vi "Config_SaveKeys.vi"(8 "error in (no error)":errorcluster, 9 "Configuration Save":T1={"General"={"Config.ini"=path "", "Default Logging Path"=path ""}, "Hardware"={"AHC VISA COM"="", "Measure Rate (1/s)"=0, "Global T VAR"="", "Global B VAR"="", "Average"=4, "Bias"=0, "Cable"={"Length"=0.0, "Resistance"=0.0, "Inductance"=0.0, "Capacitance"=0.0}, "Tracking"=0, "Voltage"=0.0}, "Operation"={"Operation Mode"=enum."Idle-Off", "Status"="", "NewLog?"=FALSE}}, 10 "Configuration Cluster":T1={"General"={"Config.ini"=path "", "Default Logging Path"=path ""}, "Hardware"={"AHC VISA COM"="", "Measure Rate (1/s)"=0, "Global T VAR"="", "Global B VAR"="", "Average"=4, "Bias"=0, "Cable"={"Length"=0.0, "Resistance"=0.0, "Inductance"=0.0, "Capacitance"=0.0}, "Tracking"=0, "Voltage"=0.0}, "Operation"={"Operation Mode"=enum."Idle-Off", "Status"="", "NewLog?"=FALSE}}, 11 "Config In":T3) -> (0 "error out":errorcluster, 2 "output cluster":T1={"General"={"Config.ini"=path "", "Default Logging Path"=path ""}, "Hardware"={"AHC VISA COM"="", "Measure Rate (1/s)"=0, "Global T VAR"="", "Global B VAR"="", "Average"=4, "Bias"=0, "Cable"={"Length"=0.0, "Resistance"=0.0, "Inductance"=0.0, "Capacitance"=0.0}, "Tracking"=0, "Voltage"=0.0}, "Operation"={"Operation Mode"=enum."Idle-Off", "Status"="", "NewLog?"=FALSE}}, 3 "refnum out":T3)   [LabVIEW 2021]
uses:
  <vilib>/Utility/config.llb/Config Data RefNum.ctl
  Config_Cluster.ctl
  Mode_Enum.ctl
  <vilib>/Utility/config.llb/Write Key (Path).vi
  <vilib>/Utility/config.llb/Write Key (String).vi
  <vilib>/Utility/config.llb/Write Key (U32).vi
  <vilib>/Utility/config.llb/Write Key (Double).vi
  <vilib>/Utility/config.llb/Write Key (I32).vi
  <vilib>/Utility/config.llb/NI_LVConfig.lvlib
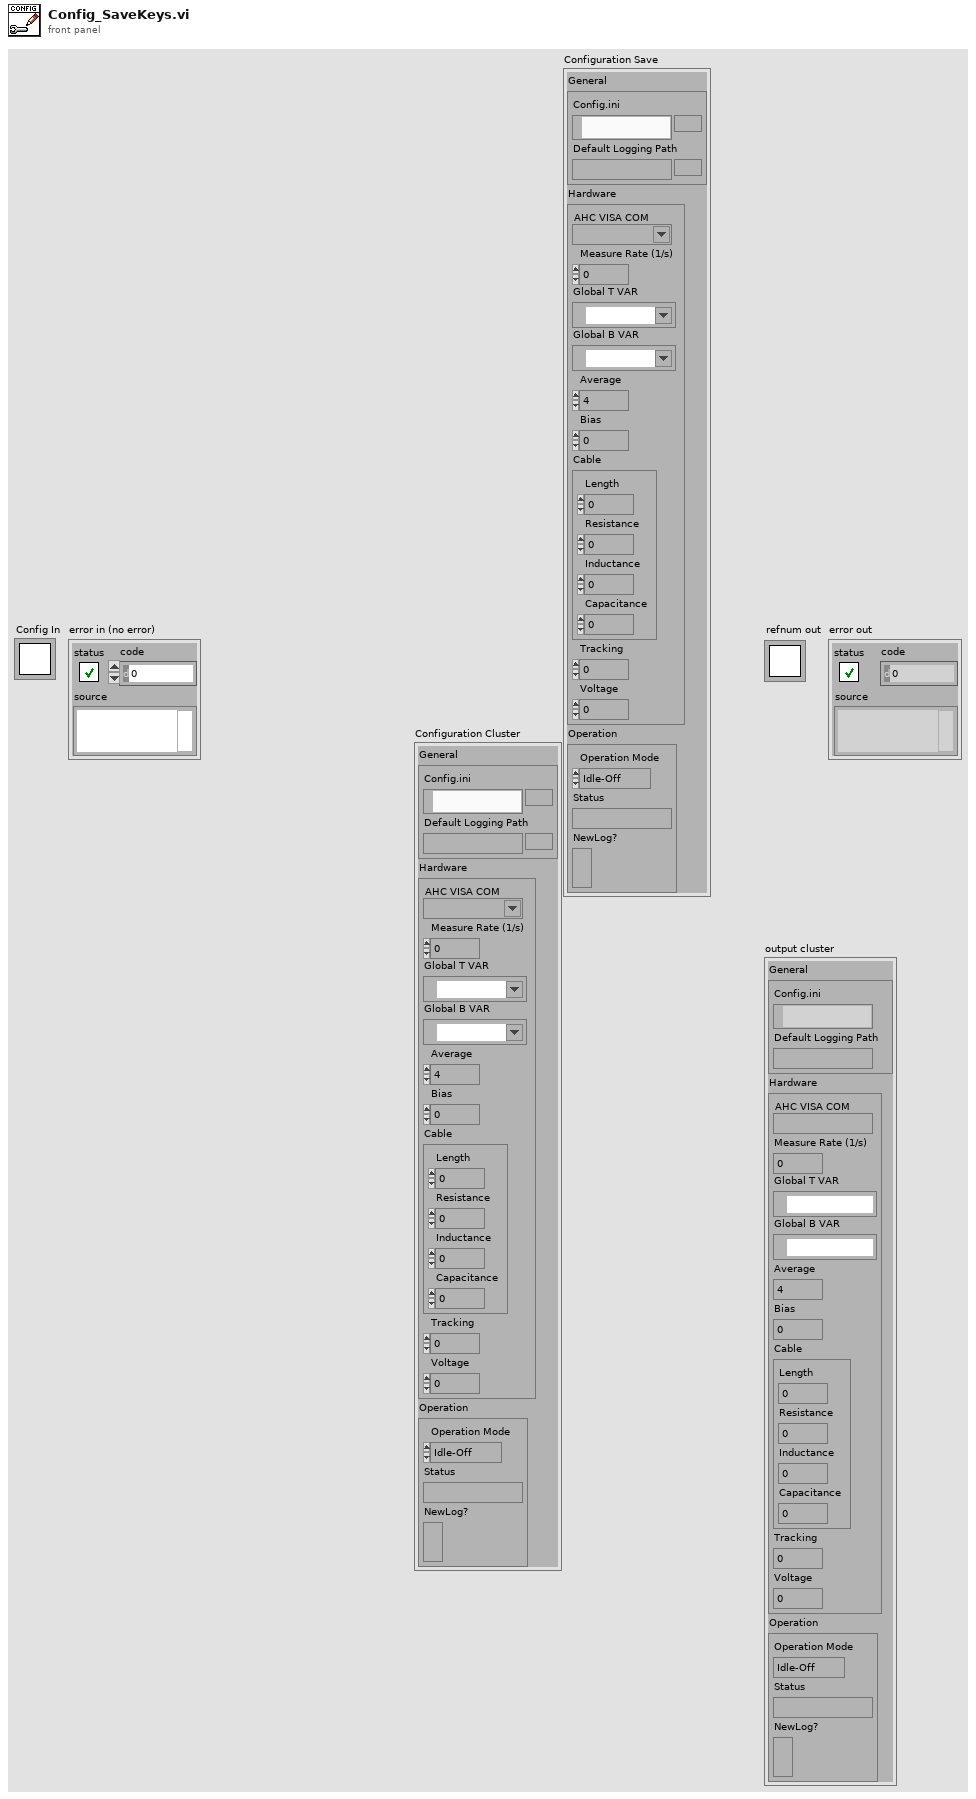
[diagram p1: front panel]
types:
  T1 = typedef "Config_Cluster.ctl" = cluster{"General":cluster{"Config.ini":path, "Default Logging Path":path}, "Hardware":cluster{"AHC VISA COM":refnum<visa-resource-name>, "Measure Rate (1/s)":i32, "Global T VAR":refnum<k21>, "Global B VAR":refnum<k21>, "Average":u8, "Bias":u8, "Cable":cluster{"Length":dbl, "Resistance":dbl, "Inductance":dbl, "Capacitance":dbl}, "Tracking":u8, "Voltage":dbl}, "Operation":cluster{"Operation Mode":T2, "Status":string, "NewLog?":bool}}
  T2 = typedef "Mode_Enum.ctl" = enum16{"Logging", "Idle-Off", "Idle"}
  T3 = typedef "NI_LVConfig.lvlib/Config Data RefNum.ctl" = refnum<k1>
  T4 = cluster{"Length":dbl, "Resistance":dbl, "Inductance":dbl, "Capacitance":dbl}
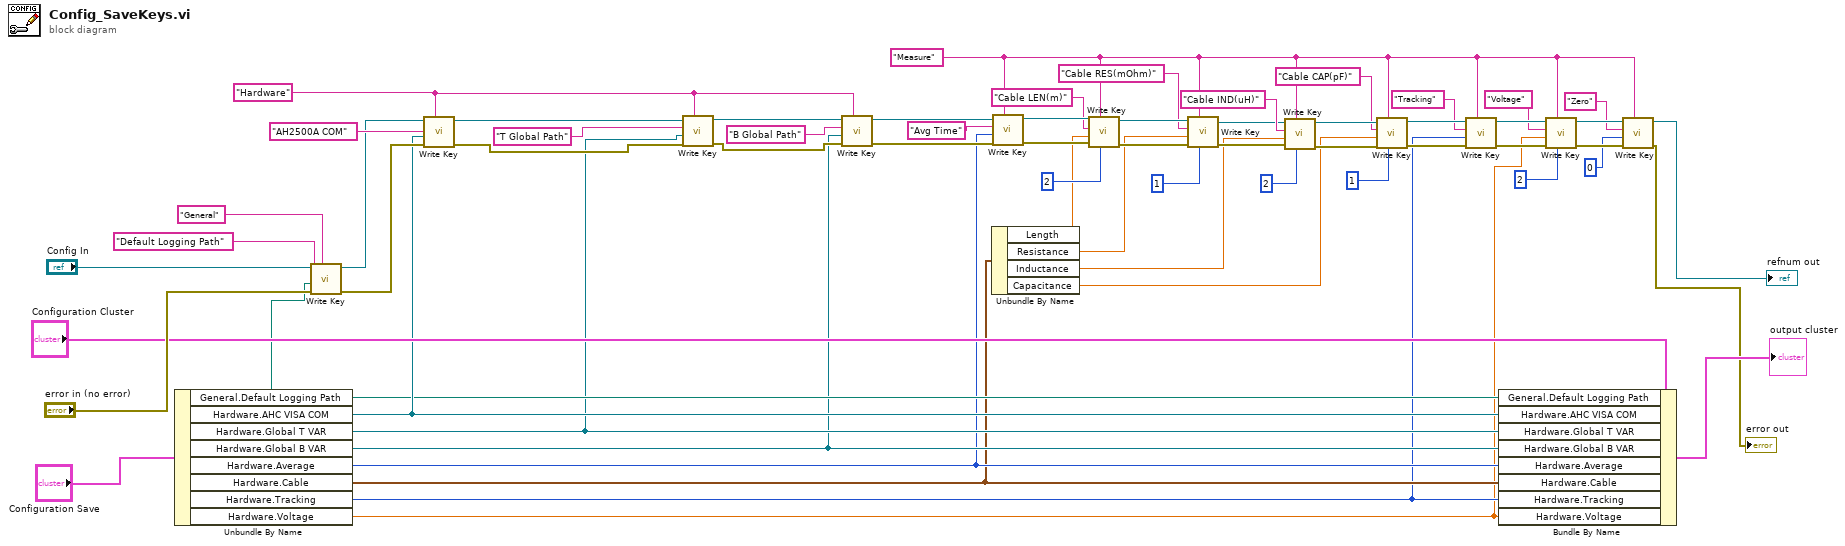
[diagram p0: block diagram]
diagram:
  w21 = "Measure" ("section")
  w52 = "Hardware" ("section")
  n1 = Unbundle By Name("Configuration Save") -> ("General.Default Logging Path"=w13:path, "Hardware.AHC VISA COM"=w14:refnum<visa-resource-name>, "Hardware.Global T VAR"=w12:refnum<k21>, "Hardware.Global B VAR"=w11:refnum<k21>, "Hardware.Average"=w10:u8, "Hardware.Cable"=w9:T4, "Hardware.Tracking"=w4:u8, "Hardware.Voltage"=w3:dbl)
  n2 = call-poly <vilib>:"Write Key.vi"("section"="General", "error in (no error)"="error in (no error)", "value"=w13, "key"="Default Logging Path", "refnum"="Config In") -> ("error out"=w16:errorcluster, "refnum out"=w17:T3)  [unwired: 4 in, 1 out]
  n3 = call-poly <vilib>:"Write Key.vi"("section"=w52, "error in (no error)"=w16, "value"=w14, "key"="AH2500A COM", "refnum"=w17) -> ("error out"=w54:errorcluster, "refnum out"=w55:T3)  [unwired: 4 in, 1 out]
  n4 = call-poly <vilib>:"Write Key.vi"("section"=w52, "error in (no error)"=w54, "value"=w12, "key"="T Global Path", "refnum"=w55) -> ("error out"=w49:errorcluster, "refnum out"=w53:T3)  [unwired: 4 in, 1 out]
  n5 = call-poly <vilib>:"Write Key.vi"("section"=w52, "error in (no error)"=w49, "value"=w11, "key"="B Global Path", "refnum"=w53) -> ("error out"=w47:errorcluster, "refnum out"=w48:T3)  [unwired: 4 in, 1 out]
  n6 = Unbundle By Name(w9) -> ("Length"=w8:dbl, "Resistance"=w7:dbl, "Inductance"=w6:dbl, "Capacitance"=w5:dbl)
  n7 = call-poly <vilib>:"Write Key.vi"("section"=w21, "error in (no error)"=w47, "value"=w10, "key"="Avg Time", "refnum"=w48) -> ("error out"=w44:errorcluster, "refnum out"=w45:T3)  [unwired: 4 in, 1 out]
  n8 = call-poly <vilib>:"Write Key.vi"("precision (6)"=i16 2, "section"=w21, "error in (no error)"=w44, "value"=w8, "key"="Cable LEN(m)", "refnum"=w45) -> ("error out"=w40:errorcluster, "refnum out"=w41:T3)  [unwired: 3 in, 1 out]
  n9 = call-poly <vilib>:"Write Key.vi"("precision (6)"=i16 1, "section"=w21, "error in (no error)"=w40, "value"=w7, "key"="Cable RES(mOhm)", "refnum"=w41) -> ("error out"=w36:errorcluster, "refnum out"=w35:T3)  [unwired: 3 in, 1 out]
  n10 = call-poly <vilib>:"Write Key.vi"("precision (6)"=i16 2, "section"=w21, "error in (no error)"=w36, "value"=w6, "key"="Cable IND(uH)", "refnum"=w35) -> ("error out"=w32:errorcluster, "refnum out"=w33:T3)  [unwired: 3 in, 1 out]
  n11 = call-poly <vilib>:"Write Key.vi"("precision (6)"=i16 1, "section"=w21, "error in (no error)"=w32, "value"=w5, "key"="Cable CAP(pF)", "refnum"=w33) -> ("error out"=w28:errorcluster, "refnum out"=w29:T3)  [unwired: 3 in, 1 out]
  n12 = call-poly <vilib>:"Write Key.vi"("section"=w21, "error in (no error)"=w28, "value"=w4, "key"="Tracking", "refnum"=w29) -> ("error out"=w25:errorcluster, "refnum out"=w26:T3)  [unwired: 4 in, 1 out]
  n13 = Bundle By Name(cluster="Configuration Cluster", "General.Default Logging Path"=w13, "Hardware.AHC VISA COM"=w14, "Hardware.Global T VAR"=w12, "Hardware.Global B VAR"=w11, "Hardware.Average"=w10, "Hardware.Cable"=w9, "Hardware.Tracking"=w4, "Hardware.Voltage"=w3) -> (→"output cluster":T1)
  n14 = call-poly <vilib>:"Write Key.vi"("precision (6)"=i16 2, "section"=w21, "error in (no error)"=w25, "value"=w3, "key"="Voltage", "refnum"=w26) -> ("error out"=w20:errorcluster, "refnum out"=w22:T3)  [unwired: 3 in, 1 out]
  n15 = call-poly <vilib>:"Write Key.vi"("section"=w21, "error in (no error)"=w20, "value"=0, "key"="Zero", "refnum"=w22) -> ("error out"=→"error out":errorcluster, "refnum out"=→"refnum out":T3)  [unwired: 4 in, 1 out]
